vi "Reserve.vi"(6 "Reply Queue":refnum<queue>, 7 "Overbook Reserve Action":enum16{"Error", "Override"}(ring), 8 "error in (no error)":errorcluster, 9 "Actor Enquerer":refnum<class "Message Enqueuer.lvclass">, 10 "Executor Number":i32, 11 "Executor":refnum<class "Executor.lvclass">) -> (0 "error out":errorcluster, 3 "Executor":refnum<class "Executor.lvclass">)   [LabVIEW 2014, in "Executor.lvclass"]
uses:
  Executor.lvclass
  <vilib>/ActorFramework/Message Enqueuer/Message Enqueuer.lvclass
  Controls/Job Results - STYP.ctl
  Executor.lvclass/Executor.ctl
  Controls/Executor Data - STYP.ctl
  Controls/Executor Status - STYP.ctl
  <vilib>/Utility/error.llb/Error Cluster From Error Code.vi
  <vilib>/ErrorRing/Error Ring.xnode
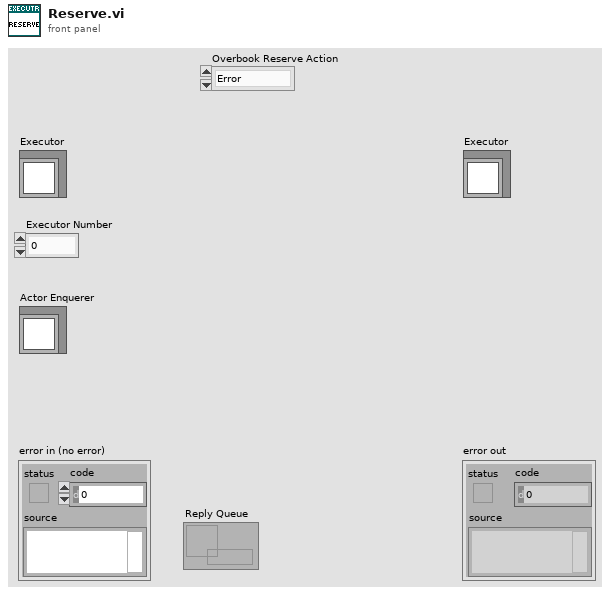
[diagram p1: front panel]
types:
  T1 = typedef "Executor Data - STYP.ctl" = cluster{"Status":T2, "Result Queue":refnum<queue>, "Actor Enquerer":refnum<class "Message Enqueuer.lvclass">}
  T2 = typedef "Executor Status - STYP.ctl" = cluster{"Executor Name":string, "Status":bool}
  T3 = typedef "Job Results - STYP.ctl" = cluster{"Status":u16, "Text":string, "Executor Number":i32}
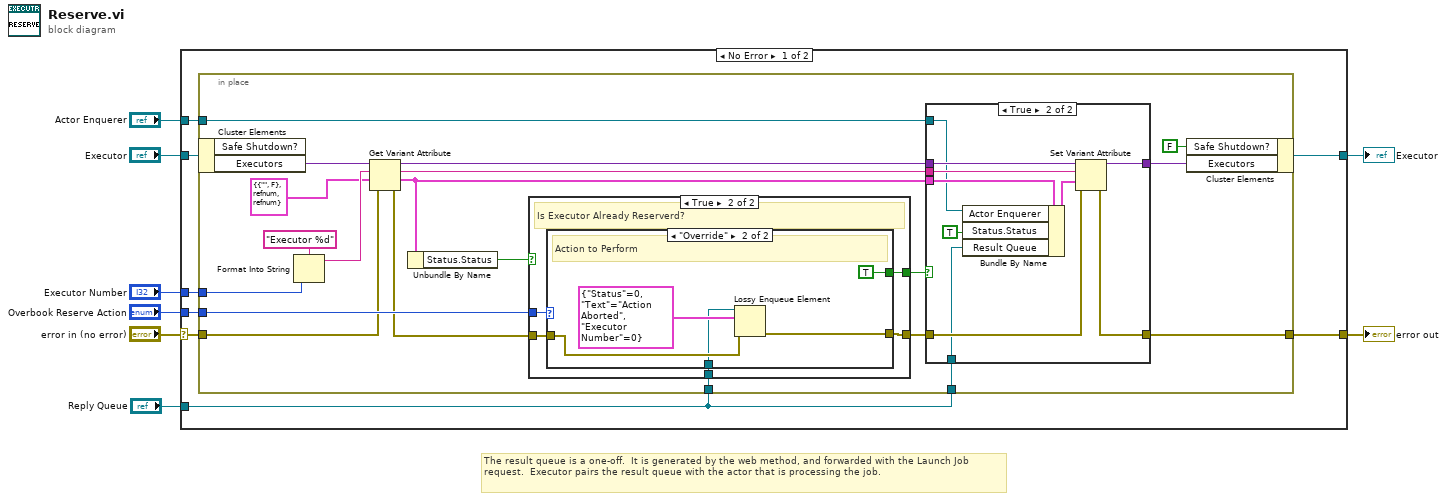
[diagram p0: block diagram]
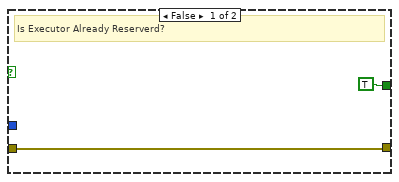
[diagram p2: hidden frame]
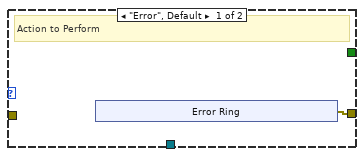
[diagram p3: hidden frame]
diagram:
  # "The result queue is a one-off.  It is generated by the web method, and forwarded with the Launch Job request.  Executor pairs the result queue with the actor that is processing the job."
  n1 = case shown="No Error" "error in (no error)" {
    selector: "error in (no error)" -> [w10 w67]
    tunnel: [w14 w67] -> w7
    tunnel: [w11 w66] -> w5
    tunnel: "Executor" -> [w12 w66]
    tunnel: "Executor Number" -> [w16 _]
    tunnel: "Overbook Reserve Action" -> [w15 _]
    tunnel: "Actor Enquerer" -> [w13 _]
    tunnel: "Reply Queue" -> [w9 _]
    frame No Error {
      n2 = in-place {
        in-place-border: w16 -> [w33]
        in-place-border: w15 -> [w25]
        in-place-border: [w27] -> w14
        in-place-border: w13 -> [w21]
        in-place-border: w10 -> [w19]
        in-place-border: w9 -> [w18]
        in-place-border: w9 -> [w17]
        n3 = in-place-cluster #1(w12) -> ("Executors"=w35:variant)  [unwired: 1 out]
        n4 = Format Into String(format string="Executor %d", w33) -> (resulting string=w32:string)  [unwired: 2 in, 1 out]
        n5 = Get Variant Attribute(Variant=w35, name=w32, default value (empty Variant)=T1 {"Status"={"Executor Name"="", "Status"=FALSE}, "Result Queue"=refnum, "Actor Enquerer"=refnum} ("Executor Data"), error in=w19) -> (duplicate Variant=w31:variant, value=w28:T1, error out=w22:errorcluster)  [unwired: 1 out]
        n6 = Unbundle By Name(w28) -> ("Status.Status"=w26:bool)
        n7 = case shown="True" w26 {
          tunnel: w25 -> [_ w42]
          tunnel: [w36 w41] -> w24
          tunnel: [TRUE w40] -> w23
          tunnel: w22 -> [w36 w39]
          tunnel: w18 -> [_ w38]
          frame False {
            # "Is Executor Already Reserverd?"
          }
          frame True {
            # "Is Executor Already Reserverd?"
            n8 = case shown="\"Override\"" w42 {
              tunnel: [w43 w51] -> w41
              tunnel: [_ TRUE] -> w40
              tunnel: w39 -> [_ w50]
              tunnel: w38 -> [_ w49]
              frame "Error", Default {
                # "Action to Perform"
                n9 = xnode "Error Ring"() -> ("error out"=w43:errorcluster)
              }
              frame "Override" {
                # "Action to Perform"
                n10 = Lossy Enqueue Element(queue=w49, element=T3 {"Status"=0, "Text"="Action Aborted", "Executor Number"=0}, error in (no error)=w50) -> (error out=w51:errorcluster)  [unwired: 3 out]
              }
            }
          }
        }
        n11 = case shown="True" w23 {
          tunnel: w32 -> [_ w63]
          tunnel: w31 -> [w55 w62]
          tunnel: [w55 w61] -> w30
          tunnel: w28 -> [_ w60]
          tunnel: [w54 w57] -> w27
          tunnel: w24 -> [w54 w59]
          tunnel: w21 -> [_ w58]
          tunnel: w17 -> [_ w56]
          frame False {
          }
          frame True {
            n12 = Bundle By Name(cluster=w60, "Actor Enquerer"=w58, "Status.Status"=TRUE ("Status"), "Result Queue"=w56) -> (w64:T1)
            n13 = Set Variant Attribute(Variant=w62, name=w63, value=w64, error in=w59) -> (Variant out=w61:variant, error out=w57:errorcluster)  [unwired: 1 out]
          }
        }
        n14 = in-place-cluster #1("Safe Shutdown?"=FALSE, "Executors"=w30) -> (w11:refnum<class "Executor.lvclass">)
      }
    }
    frame Error {
    }
  }
  "error out" <- w7
  "Executor" <- w5
